vi "NanoScanZ Stage Engine.vi"(0 "Unique Notifier Name":string, 11 "COM Port":string[](array[string])) -> ()   [LabVIEW 2020]
uses:
  Stages Controls/Stage Status.ctl
  Stages Controls/Stage Notifier Element.ctl
  Stages Controls/Stage Actions.ctl
  <vilib>/Instr/_visa.llb/VISA Configure Serial Port (Instr).vi
panel:
  out "Reply":string
  out "Device Info":string
  in  "Negative":bool
  in  "Positive":bool
  in  "Step Size (um)":dbl=1.0 min=0.0 max=10000.0
  in  "Get Pos":bool
  in  "Quit":bool
  out "Status":T1
  out "Position":dbl[](array[numeric])
  in  "Position (um)":dbl
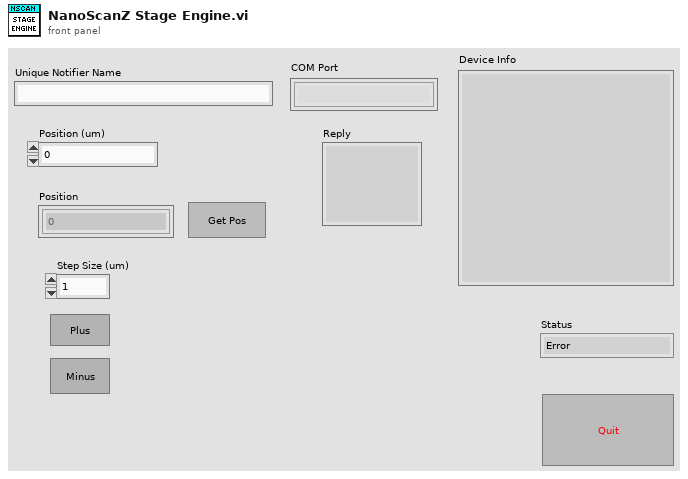
[diagram p1: front panel]
types:
  T1 = typedef "Stage Status.ctl" = enum16{"Error", "Abort", "Busy", "On Target"}
  T2 = typedef "Stage Actions.ctl" = enum16{"Get Position", "MVR", "MOVE", "HALT", "ONTARGET", "ERROR", "REFERENCE", "INIT", "VELOCITY", "STATUS", "EXIT", "HOME", "ZEROPOS", "NANOPOS", "ANALOG", "QUIT"}
  T3 = typedef "Stage Notifier Element.ctl" = cluster{"Action":T2, "Axis":bool[], "Setpoint":dbl[], "Velocity":dbl, "Cmd Recvd?":bool, "Position":dbl[], "Status":T1, "Misc":variant}
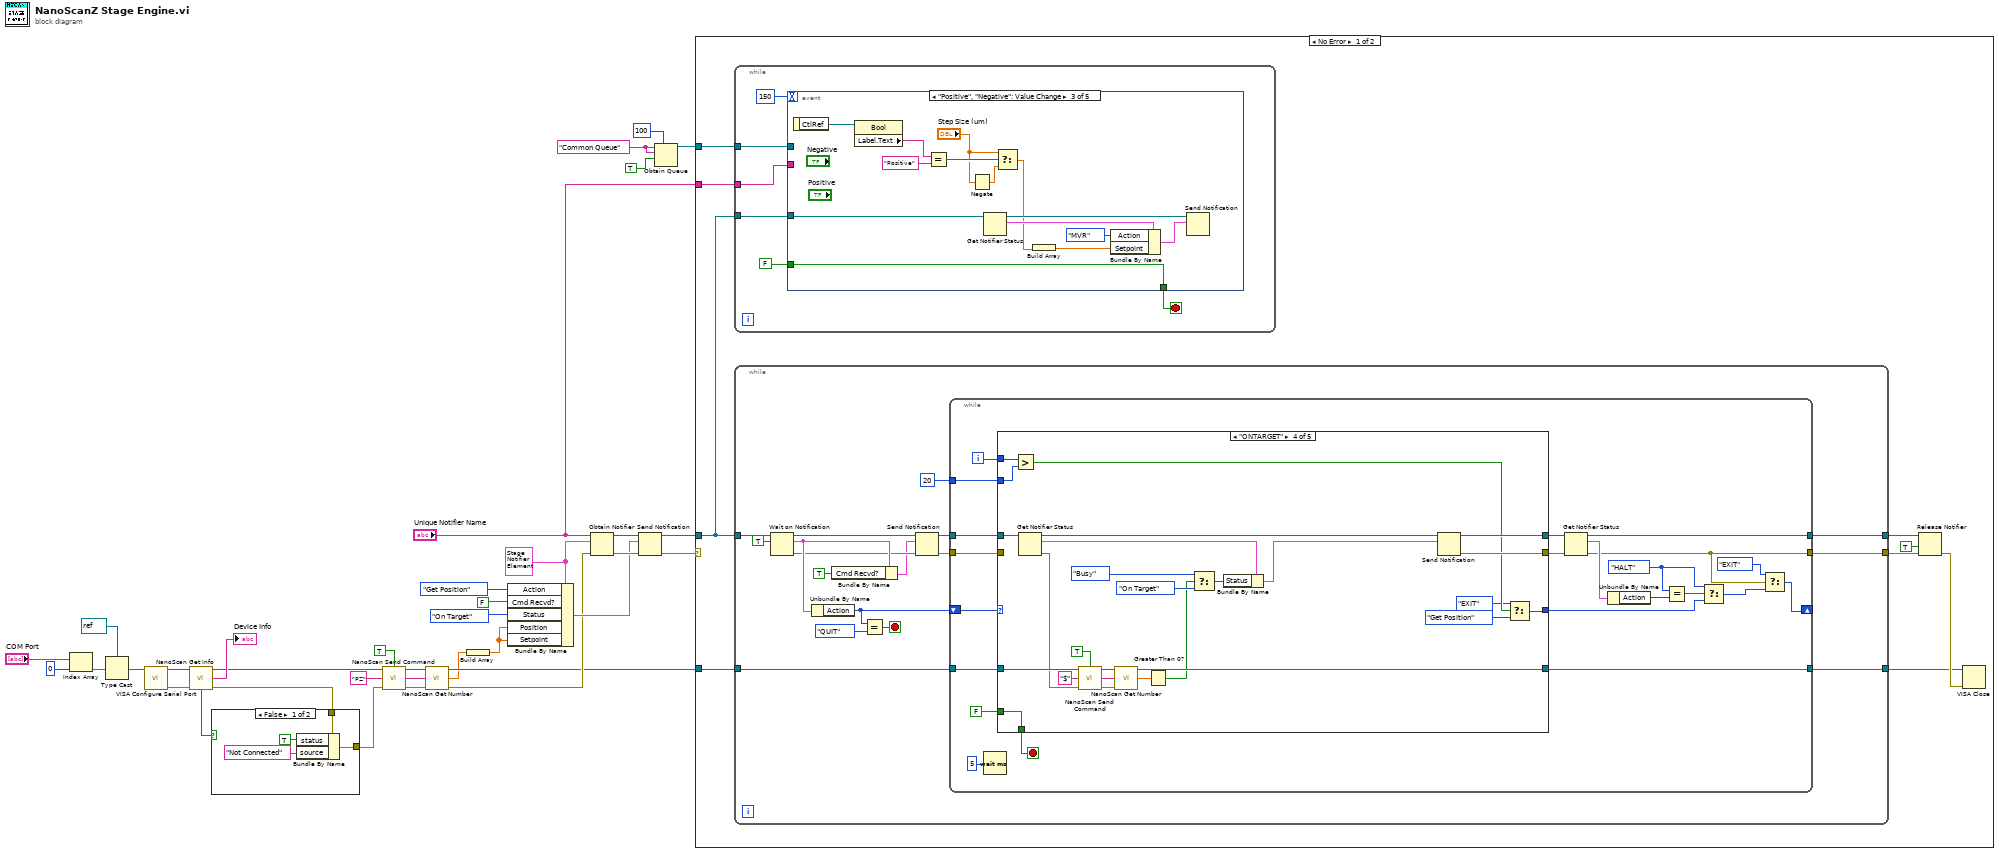
[diagram p0: block diagram]
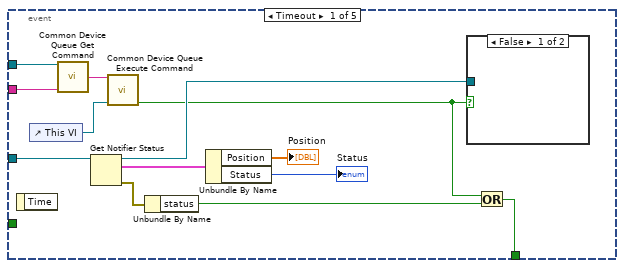
[diagram p3: hidden frame]
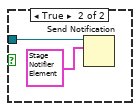
[diagram p4: hidden frame]
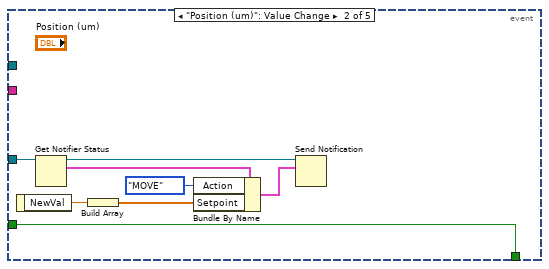
[diagram p5: hidden frame]
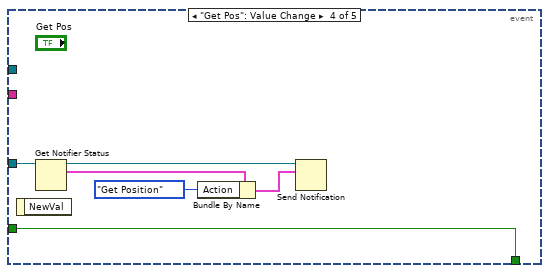
[diagram p6: hidden frame]
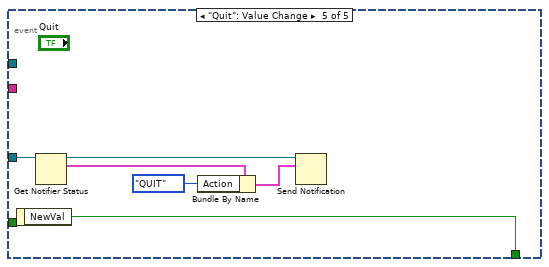
[diagram p7: hidden frame]
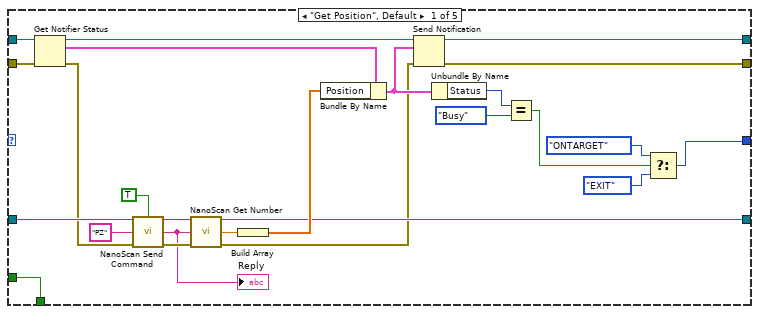
[diagram p8: hidden frame]
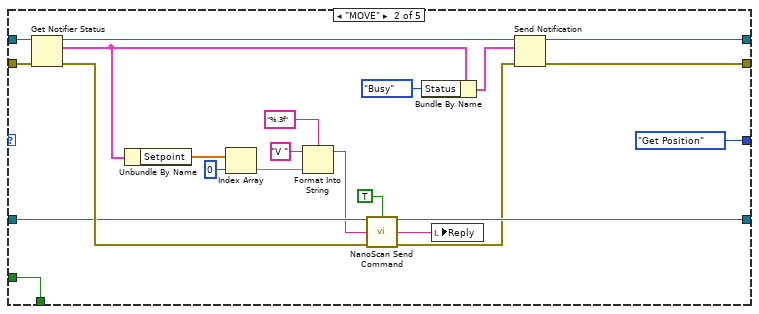
[diagram p9: hidden frame]
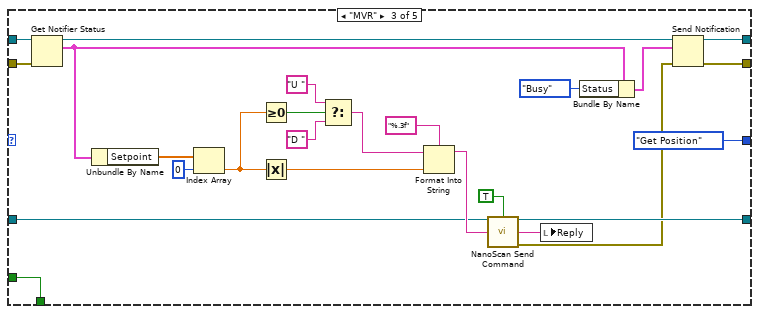
[diagram p10: hidden frame]
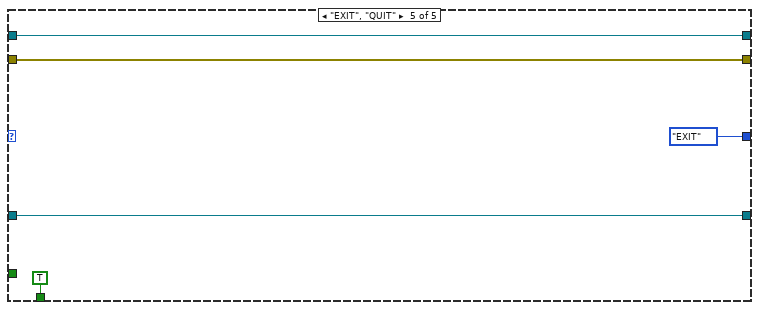
[diagram p11: hidden frame]
diagram:
  w30 = "Common Queue" ("Unique Notifier Name")
  w21 = T3 {"Action"=enum."Get Position", "Axis"=[], "Setpoint"=[], "Velocity"=0.5, "Cmd Recvd?"=FALSE, "Position"=[], "Status"=enum."Abort", "Misc"=variant} ("Stage Status")
  n1 = Index Array(array="COM Port", index=0) -> (element=w34:string)
  n2 = Type Cast(type=refnum<visa-resource-name> refnum ("reference out"), x=w34) -> (*(type *) &x=w31:refnum<visa-resource-name>)
  n3 = call-poly "VISA Configure Serial Port"("VISA resource name"=w31) -> ("VISA resource name out"=w16:refnum<visa-resource-name>, "error out"=w15:errorcluster)  [unwired: 13 in]
  n4 = call "NanoScan Get Info.vi"("VISA Ref"=w16, "Error In"=w15) -> ("VISA Ref Dup"=w11:refnum<visa-resource-name>, "Reply"=→"Device Info":string, "Connected"=w13:bool, "Error Out"=w12:errorcluster)  [unwired: 10 in]
  n5 = case shown="False" w13 {
    tunnel: w12 -> [w39 w40]
    tunnel: [w36 w40] -> w10
    frame False {
      n6 = Bundle By Name(cluster=w39, "status"=TRUE, "source"="Not Connected") -> (w36:errorcluster)
    }
    frame True {
    }
  }
  n7 = call "NanoScan Send Command.vi"("VISA Ref"=w11, "Wait for Reply (T)"=TRUE, "Command"="PZ", "Error In"=w10) -> ("VISA Ref Dup"=w6:refnum<visa-resource-name>, "Reply"=w3:string, "Error Out"=w7:errorcluster)  [unwired: 8 in, 1 out]
  n8 = call "NanoScan Get Number.vi"("VISA Ref"=w6, "Reply"=w3, "Error In"=w7) -> ("VISA Ref Dup"=w4:refnum<visa-resource-name>, "Number"=w2:dbl, "Error Out"=w5:errorcluster)  [unwired: 10 in]
  n9 = Build Array(w2) -> (w1:dbl[])
  n10 = Bundle By Name(cluster=w21, "Action"=Stage_Actions."Get Position", "Cmd Recvd?"=FALSE, "Status"=Stage_Status."On Target", "Position"=w1, "Setpoint"=w1) -> (w22:T3)
  n11 = Obtain Notifier(name (unnamed)="Unique Notifier Name", notification data type=w21, error in (no error)=w5) -> (notifier out=w25:refnum<notifier>, error out=w24:errorcluster)  [unwired: 1 in, 1 out]
  n12 = Send Notification(notification=w22, notifier=w25, error in (no error)=w24) -> (notifier out=w18:refnum<notifier>, error out=w17:errorcluster)
  n13 = Obtain Queue(max queue size (-1, unlimited)=100, name (unnamed)=w30, element data type=w30, create if not found? (T)=TRUE) -> (queue out=w26:refnum<queue>)  [unwired: 1 in, 2 out]
  n14 = case shown="No Error" w17 {
    tunnel: w4 -> [w49 _]
    tunnel: w18 -> [w41 _]
    tunnel: "Unique Notifier Name" -> [w44 _]
    tunnel: w26 -> [w43 _]
    frame No Error {
      n15 = while {
        tunnel: w44 -> [w53]
        tunnel: w43 -> [w54]
        tunnel: w41 -> [w52]
        stop <- w51 stop-if-true
        n16 = event shown="[2] \"Positive\", \"Negative\": Value Change" {
          selector: _ -> [_ _ _ _ _]
          dyn-events: _ -> [_ _ _ _ _]
          timeout: 150 -> [_ _ _ _ _]
          tunnel: w54 -> [w66 _ _ _ _]
          tunnel: w53 -> [w65 _ _ _ _]
          tunnel: w52 -> [w64 w77 w80 w97 w104]
          tunnel: [w58 w78 w92 w98 w99] -> w51
          tunnel: FALSE -> [_ w78 w92 w98 _]
          event Timeout {
            n17 = event-data() -> ()  [unwired: 1 in, 1 out]
            n18 = control-ref of="This VI"() -> (w67:refnum<vi>)
            n19 = call "Common Device Queue Get Command.vi"("Common Queue"=w66, "Notifier Name"=w65) -> ("Command"=w68:string)  [unwired: 12 in, 1 out]
            n20 = Get Notifier Status(notifier=w64) -> (notifier out=w60:refnum<notifier>, current notification=w63:T3, error out=w62:errorcluster)  [unwired: 1 in, 2 out]
            n21 = call "Common Device Queue Execute Command.vi"("Common Command"=w68, "VI Refnum"=w67) -> ("Quit?"=w59:bool)  [unwired: 12 in, 1 out]
            n22 = Unbundle By Name(w62) -> ("status"=w61:bool)
            n23 = Unbundle By Name(w63) -> ("Position"=→"Position":dbl[], "Status"=→"Status":T1)
            n24 = case shown="False" w59 {
              tunnel: w60 -> [_ w69]
              frame False {
              }
              frame True {
                n25 = Send Notification(notification=T3 {"Action"=enum."QUIT", "Axis"=[], "Setpoint"=[], "Velocity"=0.5, "Cmd Recvd?"=FALSE, "Position"=[], "Status"=enum."Error", "Misc"=variant} ("Stage Status"), notifier=w69) -> ()  [unwired: 1 in, 2 out]
              }
            }
            n26 = Or(x=w59, y=w61) -> (x .or. y?=w58:bool)
          }
          event "Position (um)": Value Change {
            n27 = event-data() -> ("NewVal"=w72:dbl)  [unwired: 1 in]
            n28 = Get Notifier Status(notifier=w77) -> (notifier out=w75:refnum<notifier>, current notification=w76:T3)  [unwired: 1 in, 3 out]
            n29 = Build Array(w72) -> (w73:dbl[])
            n30 = Bundle By Name(cluster=w76, "Action"=Stage_Actions."MOVE", "Setpoint"=w73) -> (w74:T3)
            n31 = Send Notification(notification=w74, notifier=w75) -> ()  [unwired: 1 in, 2 out]
          }
          event "Positive", "Negative": Value Change {
            n32 = event-data() -> ("CtlRef"=w91:refnum<vi>)  [unwired: 1 in]
            n33 = property class="Bool"(reference=w91) -> ("Label.Text"=w90:string)  [unwired: 1 in, 2 out]
            n34 = Equal?(x=w90, y="Positive") -> (x = y?=w88:bool)
            n35 = Negate(x="Step Size (um)") -> (-x=w86:dbl)
            n36 = Get Notifier Status(notifier=w80) -> (notifier out=w84:refnum<notifier>, current notification=w85:T3)  [unwired: 1 in, 3 out]
            n37 = Select(t="Step Size (um)", s=w88, f=w86) -> (s? t:f=w79:dbl)
            n38 = Build Array(w79) -> (w82:dbl[])
            n39 = Bundle By Name(cluster=w85, "Action"=Stage_Actions."MVR", "Setpoint"=w82) -> (w83:T3)
            n40 = Send Notification(notification=w83, notifier=w84) -> ()  [unwired: 1 in, 2 out]
          }
          event "Get Pos": Value Change {
            n41 = event-data() -> ()  [unwired: 1 in, 1 out]
            n42 = Get Notifier Status(notifier=w97) -> (notifier out=w95:refnum<notifier>, current notification=w96:T3)  [unwired: 1 in, 3 out]
            n43 = Bundle By Name(cluster=w96, "Action"=Stage_Actions."Get Position") -> (w94:T3)
            n44 = Send Notification(notification=w94, notifier=w95) -> ()  [unwired: 1 in, 2 out]
          }
          event "Quit": Value Change {
            n45 = event-data() -> ("NewVal"=w99:bool)  [unwired: 1 in]
            n46 = Get Notifier Status(notifier=w104) -> (notifier out=w102:refnum<notifier>, current notification=w103:T3)  [unwired: 1 in, 3 out]
            n47 = Bundle By Name(cluster=w103, "Action"=Stage_Actions."QUIT") -> (w101:T3)
            n48 = Send Notification(notification=w101, notifier=w102) -> ()  [unwired: 1 in, 2 out]
          }
        }
      }
      n49 = while {
        tunnel: w41 -> [w121]
        tunnel: w49 -> [w116]
        tunnel: [w108] -> w46
        tunnel: [w107] -> w47
        tunnel: [w106] -> w45
        stop <- w118 stop-if-true
        n50 = Wait on Notification(notifier=w121, ignore previous (F)=TRUE) -> (notifier out=w112:refnum<notifier>, notification=w115:T3, error out=w113:errorcluster)  [unwired: 2 in, 1 out]
        n51 = Unbundle By Name(w115) -> ("Action"=w117:T2)
        n52 = Bundle By Name(cluster=w115, "Cmd Recvd?"=TRUE) -> (w111:T3)
        n53 = Equal?(x=w117, y=Stage_Actions."QUIT") -> (x = y?=w118:bool)
        n54 = Send Notification(notification=w111, notifier=w112, error in (no error)=w113) -> (notifier out=w109:refnum<notifier>, error out=w110:errorcluster)
        n55 = while {
          shift-right: [w128] -> _
          shift-left: w117 -> [w143]
          tunnel: w109 -> [w142]
          tunnel: w110 -> [w140]
          tunnel: w116 -> [w141]
          tunnel: [w125] -> w108
          tunnel: [w124] -> w107
          tunnel: [w123] -> w106
          tunnel: 20 -> [w122]
          i -> [w126]
          stop <- w138 stop-if-true
          w132 = Stage_Actions."HALT" ("Action")
          n56 = Wait (ms)(milliseconds to wait=u32 5) -> ()  [unwired: 1 out]
          n57 = case shown="\"ONTARGET\"" w143 {
            tunnel: w142 -> [w167 w190 w215 w227 w245]
            tunnel: w141 -> [w149 w180 w202 w224 w242]
            tunnel: w140 -> [w166 w189 w214 _ w243]
            tunnel: FALSE -> [w168 w188 w207 w232 _]
            tunnel: [w168 w188 w207 w232 TRUE] -> w138
            tunnel: w122 -> [_ _ _ w233 _]
            tunnel: [w154 Stage_Actions."Get Position" ("Action") Stage_Actions."Get Position" ("Action") w230 Stage_Actions."EXIT" ("Action")] -> w130
            tunnel: [w161 w171 w208 w240 w245] -> w136
            tunnel: [w162 w169 w193 w239 w243] -> w135
            tunnel: w126 -> [_ _ _ w234 _]
            tunnel: [w148 w178 w194 w219 w242] -> w123
            frame "Get Position", Default {
              n58 = Get Notifier Status(notifier=w167, error in (no error)=w166) -> (notifier out=w165:refnum<notifier>, current notification=w164:T3, error out=w146:errorcluster)  [unwired: 2 out]
              n59 = call "NanoScan Send Command.vi"("VISA Ref"=w149, "Wait for Reply (T)"=TRUE, "Command"="PZ", "Error In"=w146) -> ("VISA Ref Dup"=w152:refnum<visa-resource-name>, "Reply"=w144:string, "Error Out"=w153:errorcluster)  [unwired: 8 in, 1 out]
              "Reply" <- w144
              n60 = call "NanoScan Get Number.vi"("VISA Ref"=w152, "Reply"=w144, "Error In"=w153) -> ("VISA Ref Dup"=w148:refnum<visa-resource-name>, "Number"=w145:dbl, "Error Out"=w147:errorcluster)  [unwired: 10 in]
              n61 = Build Array(w145) -> (w163:dbl[])
              n62 = Bundle By Name(cluster=w164, "Position"=w163) -> (w160:T3)
              n63 = Send Notification(notification=w160, notifier=w165, error in (no error)=w147) -> (notifier out=w161:refnum<notifier>, error out=w162:errorcluster)
              n64 = Unbundle By Name(w160) -> ("Status"=w159:T1)
              n65 = Equal?(x=w159, y=Stage_Status."Busy") -> (x = y?=w157:bool)
              n66 = Select(t=Stage_Actions."ONTARGET" ("Action"), s=w157, f=Stage_Actions."EXIT" ("Action")) -> (s? t:f=w154:T2)
            }
            frame "MOVE" {
              n67 = Get Notifier Status(notifier=w190, error in (no error)=w189) -> (notifier out=w173:refnum<notifier>, current notification=w172:T3, error out=w181:errorcluster)  [unwired: 2 out]
              n68 = Unbundle By Name(w172) -> ("Setpoint"=w186:dbl[])
              n69 = Index Array(array=w186, index=0) -> (element=w184:dbl)
              n70 = Format Into String(format string="%.3f", initial string="V ", w184) -> (resulting string=w179:string)  [unwired: 1 in, 1 out]
              n71 = call "NanoScan Send Command.vi"("VISA Ref"=w180, "Wait for Reply (T)"=TRUE, "Command"=w179, "Error In"=w181) -> ("VISA Ref Dup"=w178:refnum<visa-resource-name>, "Reply"=w176:string, "Error Out"=w170:errorcluster)  [unwired: 8 in, 1 out]
              n72 = Bundle By Name(cluster=w172, "Status"=Stage_Status."Busy") -> (w175:T3)
              n73 = local write "Reply"(w176) -> ()
              n74 = Send Notification(notification=w175, notifier=w173, error in (no error)=w170) -> (notifier out=w171:refnum<notifier>, error out=w169:errorcluster)
            }
            frame "MVR" {
              n75 = Get Notifier Status(notifier=w215, error in (no error)=w214) -> (notifier out=w210:refnum<notifier>, current notification=w212:T3)  [unwired: 3 out]
              n76 = Unbundle By Name(w212) -> ("Setpoint"=w201:dbl[])
              n77 = Index Array(array=w201, index=0) -> (element=w200:dbl)
              n78 = Greater Or Equal To 0?(x=w200) -> (x >= 0?=w198:bool)
              n79 = Absolute Value(x=w200) -> (abs(x)=w199:dbl)
              n80 = Select(t="U ", s=w198, f="D ") -> (s? t:f=w195:string)
              n81 = Format Into String(format string="%.3f", initial string=w195, w199) -> (resulting string=w204:string)  [unwired: 1 in, 1 out]
              n82 = call "NanoScan Send Command.vi"("VISA Ref"=w202, "Wait for Reply (T)"=TRUE, "Command"=w204) -> ("VISA Ref Dup"=w194:refnum<visa-resource-name>, "Reply"=w191:string, "Error Out"=w192:errorcluster)  [unwired: 9 in, 1 out]
              n83 = local write "Reply"(w191) -> ()
              n84 = Bundle By Name(cluster=w212, "Status"=Stage_Status."Busy") -> (w209:T3)
              n85 = Send Notification(notification=w209, notifier=w210, error in (no error)=w192) -> (notifier out=w208:refnum<notifier>, error out=w193:errorcluster)
            }
            frame "ONTARGET" {
              n86 = Greater?(x=w234, y=w233) -> (0:w229:bool)
              n87 = Get Notifier Status(notifier=w227) -> (notifier out=w241:refnum<notifier>, current notification=w226:T3, error out=w222:errorcluster)  [unwired: 1 in, 2 out]
              n88 = call "NanoScan Send Command.vi"("VISA Ref"=w224, "Wait for Reply (T)"=TRUE, "Command"="$", "Error In"=w222) -> ("VISA Ref Dup"=w220:refnum<visa-resource-name>, "Reply"=w221:string, "Error Out"=w218:errorcluster)  [unwired: 8 in, 1 out]
              n89 = call "NanoScan Get Number.vi"("VISA Ref"=w220, "Reply"=w221, "Error In"=w218) -> ("VISA Ref Dup"=w219:refnum<visa-resource-name>, "Number"=w217:dbl)  [unwired: 10 in, 1 out]
              n90 = Greater Than 0?(x=w217) -> (x > 0?=w216:bool)
              n91 = Select(t=Stage_Status."Busy" ("Status"), s=w216, f=Stage_Status."On Target" ("Status")) -> (s? t:f=w235:T1)
              n92 = Bundle By Name(cluster=w226, "Status"=w235) -> (w238:T3)
              n93 = Send Notification(notification=w238, notifier=w241) -> (notifier out=w240:refnum<notifier>, error out=w239:errorcluster)  [unwired: 1 in]
              n94 = Select(t=Stage_Actions."EXIT", s=w229, f=Stage_Actions."Get Position" ("Action")) -> (s? t:f=w230:T2)
            }
            frame "EXIT", "QUIT" {
            }
          }
          n95 = Get Notifier Status(notifier=w136, error in (no error)=w135) -> (notifier out=w125:refnum<notifier>, current notification=w131:T3, error out=w124:errorcluster)  [unwired: 2 out]
          n96 = Unbundle By Name(w131) -> ("Action"=w133:T2)
          n97 = Equal?(x=w132, y=w133) -> (x = y?=w134:bool)
          n98 = Select(t=w132, s=w134, f=w130) -> (s? t:f=w129:T2)
          n99 = Select(t=Stage_Actions."EXIT", s=w124, f=w129) -> (s? t:f=w128:T2)
        }
      }
      n100 = Release Notifier(notifier=w46, force destroy? (F)=TRUE, error in (no error)=w47) -> (error out=w48:errorcluster)  [unwired: 2 out]
      n101 = VISA Close(VISA resource name=w45, error in (no error)=w48) -> ()  [unwired: 1 out]
    }
    frame Error {
    }
  }
